vi "Set Percentage.vi"(8 "error in (no error)":errorcluster, 9 "Right Percentage":dbl min=-1.0 max=1.0, 10 "Left Percentage":dbl min=-1.0 max=1.0, 11 "Forward Drive in":refnum<class "Forward Drive.lvclass">) -> (0 "error out":errorcluster, 3 "Forward Drive out":refnum<class "Forward Drive.lvclass">)   [LabVIEW 2014, in "Forward Drive.lvlib" / "Forward Drive.lvclass"]
uses:
  Forward Drive.lvclass
  Forward Drive.lvclass/Forward Drive.ctl
  Motor with Encoders/Motors with Encoders Messages/Set VBus Percent Msg/Set VBus Percent Msg.lvclass/Set VBus Percent Msg.ctl
  <vilib>/ActorFramework/Message Enqueuer/Message Enqueuer.lvclass/Message Enqueuer.ctl
  Motor with Encoders/Motors with Encoders Messages/Set Rate (Percent) Msg/Set Rate (Percent) Msg.lvclass/Set Rate (Percent) Msg.ctl
  <vilib>/ActorFramework/Message Enqueuer/Enqueue.vi
  <vilib>/ActorFramework/Message Priority Queue/Priority Enqueue.vi
  Motor with Encoders/Motors with Encoders Messages/Set VBus Percent Msg/Set VBus Percent Msg.lvclass
  Motor with Encoders/Motors with Encoders Messages/Set Rate (Percent) Msg/Set Rate (Percent) Msg.lvclass
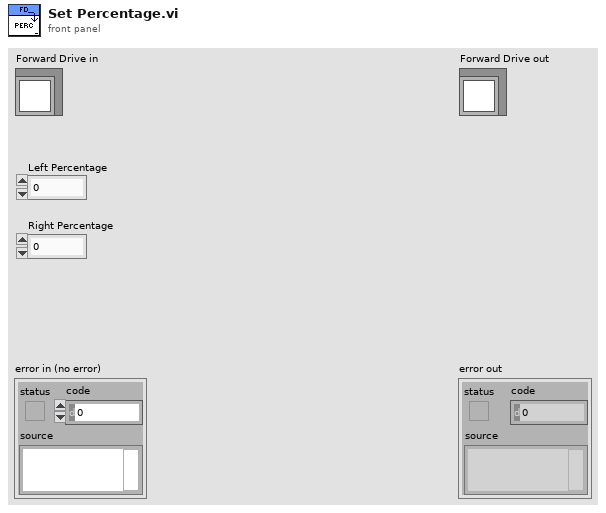
[diagram p1: front panel]
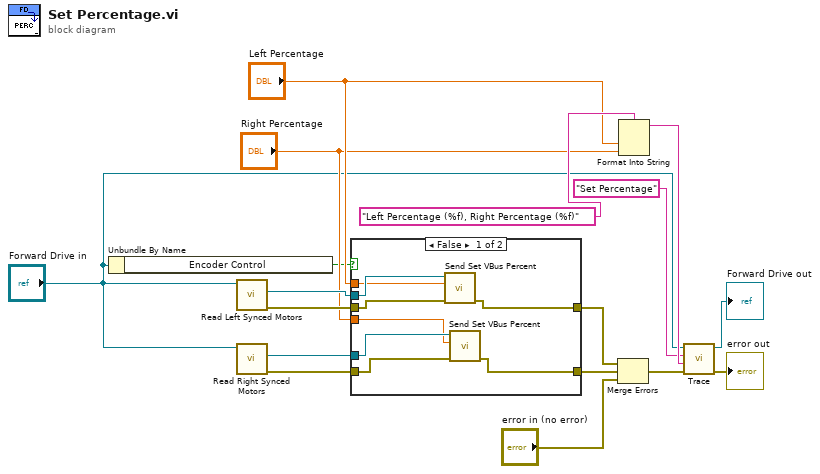
[diagram p0: block diagram]
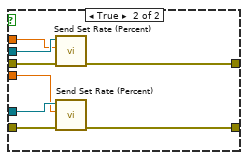
[diagram p2: hidden frame]
diagram:
  n1 = Unbundle By Name("Forward Drive in") -> ("Encoder Control"=w1:bool)
  n2 = call-dynamic "Read Left Synced Motors.vi"("Forward Drive in"="Forward Drive in") -> ("error out"=w10:errorcluster, "Actor Framework:Message Enqueuer"=w9:refnum<class "Message Enqueuer.lvclass">)  [unwired: 8 in, 1 out]
  n3 = call-dynamic "Read Right Synced Motors.vi"("Forward Drive in"="Forward Drive in") -> ("error out"=w11:errorcluster, "Actor Framework:Message Enqueuer"=w6:refnum<class "Message Enqueuer.lvclass">)  [unwired: 8 in, 1 out]
  n4 = case shown="False" w1 {
    tunnel: [w18 w33] -> w13
    tunnel: [w20 w32] -> w12
    tunnel: w11 -> [w19 w31]
    tunnel: w10 -> [w21 w30]
    tunnel: w9 -> [w25 w29]
    tunnel: "Left Percentage" -> [w24 w28]
    tunnel: w6 -> [w23 w27]
    tunnel: "Right Percentage" -> [w22 w26]
    frame False {
      n5 = call "Send Set VBus Percent.vi"("error in (no error)"=w21, "Percent VBus"=w24, "Message Enqueuer"=w25) -> ("error out"=w20:errorcluster)  [unwired: 7 in, 1 out]
      n6 = call "Send Set VBus Percent.vi"("error in (no error)"=w19, "Percent VBus"=w22, "Message Enqueuer"=w23) -> ("error out"=w18:errorcluster)  [unwired: 7 in, 1 out]
    }
    frame True {
      n7 = call "Send Set Rate (Percent).vi"("error in (no error)"=w30, "Rate (Percentage)"=w28, "Message Enqueuer"=w29) -> ("error out"=w32:errorcluster)  [unwired: 7 in, 1 out]
      n8 = call "Send Set Rate (Percent).vi"("error in (no error)"=w31, "Rate (Percentage)"=w26, "Message Enqueuer"=w27) -> ("error out"=w33:errorcluster)  [unwired: 7 in, 1 out]
    }
  }
  n9 = Merge Errors(w12, w13, "error in (no error)") -> (w15:errorcluster)
  n10 = Format Into String(format string="Left Percentage (%f), Right Percentage (%f)", "Left Percentage", "Right Percentage") -> (resulting string=w4:string)  [unwired: 2 in, 1 out]
  n11 = call-dynamic "Trace.vi"("error in (no error)"=w15, "System Message"=w4, "System Action"="Set Percentage", "System Actor in"="Forward Drive in") -> ("error out"=→"error out":errorcluster, "System Actor out"=→"Forward Drive out":refnum<class "Forward Drive.lvclass">)  [unwired: 6 in]
